vi "Get Decoration Label.vi"(4 "error in":errorcluster, 7 "Decor Refnum":refnum<vi>) -> (0 "error out":errorcluster, 2 "Label":string, 3 "dup Decor Refnum":refnum<vi>)   [LabVIEW 2020]
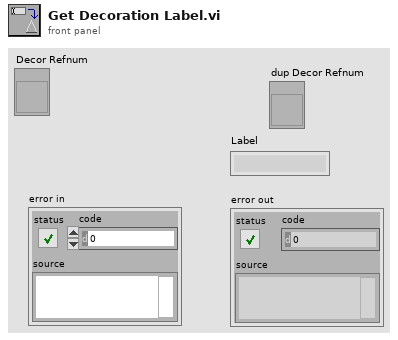
[diagram p1: front panel]
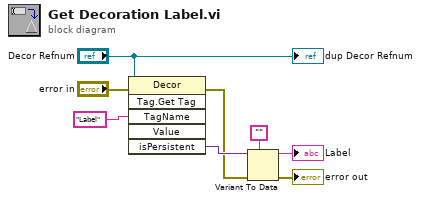
[diagram p0: block diagram]
diagram:
  n1 = invoke class="Decor" method="Tag.Get Tag"(reference="Decor Refnum", error in="error in", "TagName"="Label" ("Tag Name")) -> (error out=w4:errorcluster, "isPersistent"=w5:variant)  [unwired: 3 in, 4 out]
  n2 = Variant To Data(error in=w4, type="", Variant=w5) -> (data=→"Label":string, error out=→"error out":errorcluster)
  "dup Decor Refnum" <- "Decor Refnum"
